vi "Func-Hex array string to bin file.vi"() -> ()   [LabVIEW 2015]
panel:
  out "array 2d":u8[][](array[numeric])=[[27, 0, 0, 0, 0, 0, 0, 0, 0, 0, 1, 56, 33, 80, 255, 239], [240, 93, 1, 0, 0, 0, 6, 1, 1, 165, 16, 0, 0, 2, 2, 2], [4, 4, 4, 4, 4, 4, 4, 0, 33, 191, 136, 2, 32, 32, 160, 132], [0, 6, 46, 47, 7, 211, 145, 27, 40, 68, 0, 10, 15, 0, 15, 108], [204, 91, 248, 23, 35, 154, 71, 0, 48, 24, 22, 108, 3, 96, 145, 2], [14, 120, 86, 16, 234, 42, 0, 31, 65, 0, 0, 0, 205, 124, 10, 137], [6, 8, 8, 3, 245, 0, 0, 39, 15, 128, 0, 128, 0, 0, 0, 0], [0, 255, 100, 100, 24, 1, 137, 6, 8, 8, 3, 245, 0, 0, 39, 15], [128, 0, 128, 0, 0, 0, 0, 0, 255, 100, 100, 24, 2, 137, 6, 8], [8, 3, 245, 0, 0, 39, 15, 128, 0, 128, 0, 0, 0, 0, 0, 255], [100, 100, 24, 3, 137, 6, 8, 8, 3, 245, 0, 0, 39, 15, 128, 0], [128, 0, 0, 0, 0, 0, 255, 100, 100, 24, 4, 137, 6, 8, 8, 3], [245, 0, 0, 39, 15, 128, 0, 128, 0, 0, 0, 0, 0, 255, 100, 100], [24, 5, 137, 6, 8, 8, 3, 245, 0, 0, 39, 15, 128, 0, 128, 0], [0, 0, 0, 0, 255, 100, 100, 24, 6, 137, 6, 8, 8, 3, 245, 0], [0, 39, 15, 128, 0, 128, 0, 0, 0, 0, 0, 255, 100, 100, 24, 7], [137, 6, 8, 8, 3, 245, 0, 0, 39, 15, 128, 0, 128, 0, 0, 0], [0, 0, 255, 100, 100, 24, 8, 137, 6, 8, 8, 3, 245, 0, 0, 39], [15, 128, 0, 128, 0, 0, 0, 0, 0, 255, 100, 100, 24, 9, 137, 6], [8, 8, 3, 245, 0, 0, 39, 15, 128, 0, 128, 0, 0, 0, 0, 0], [255, 100, 100, 24, 10, 137, 6, 8, 8, 3, 245, 0, 0, 39, 15, 128], [0, 128, 0, 0, 0, 0, 0, 255, 100, 100, 24, 11, 137, 6, 8, 8], [3, 245, 0, 0, 39, 15, 128, 0, 128, 0, 0, 0, 0, 0, 255, 100], [100, 24, 12, 137, 6, 8, 8, 3, 245, 0, 0, 39, 15, 128, 0, 128], [0, 0, 0, 0, 0, 255, 100, 100, 24, 13, 137, 6, 8, 8, 3, 245], [0, 0, 39, 15, 128, 0, 128, 0, 0, 0, 0, 0, 255, 100, 100, 24], [14, 137, 6, 8, 8, 3, 245, 0, 0, 39, 15, 128, 0, 128, 0, 0], [0, 0, 0, 255, 100, 100, 24, 15, 137, 6, 8, 8, 3, 245, 0, 0], [39, 15, 128, 0, 128, 0, 0, 0, 0, 0, 255, 100, 100, 24, 16, 137], [6, 8, 8, 3, 245, 0, 0, 39, 15, 128, 0, 128, 0, 0, 0, 0], [0, 255, 100, 100, 24, 17, 137, 6, 8, 8, 3, 245, 0, 0, 39, 15], [128, 0, 128, 0, 0, 0, 0, 0, 255, 100, 100, 24, 18, 128, 0, 0]] format="%02x"
  in  "Hex array string":string="1B\t00\t00\t00\t00\t00\t00\t00\t00\t00\t01\t38\t21\t50\tFF\tEF\nF0\t5D\t01\t00\t00\t00\t06\t01\t01\tA5\t10\t00\t00\t02\t02\t02\n04\t04\t04\t04\t04\t04\t04\t00\t21\tBF\t88\t02\t20\t20\tA0\t84\n00\t06\t2E\t2F\t07\tD3\t91\t1B\t28\t44\t00\t0A\t0F\t00\t0F\t6C\nCC\t5B\tF8\t17\t23\t9A\t47\t00\t30\t18\t16\t6C\t03\t60\t91\t02\n0E\t78\t56\t10\tEA\t2A\t00\t1F\t41\t00\t00\t00\tCD\t7C\t0A\t89\n06\t08\t08\t03\tF5\t00\t00\t27\t0F\t80\t00\t80\t00\t00\t00\t00\n00\tFF\t64\t64\t18\t01\t89\t06\t08\t08\t03\tF5\t00\t00\t27\t0F\n80\t00\t80\t00\t00\t00\t00\t00\tFF\t64\t64\t18\t02\t89\t06\t08\n08\t03\tF5\t00\t00\t27\t0F\t80\t00\t80\t00\t00\t00\t00\t00\tFF\n64\t64\t18\t03\t89\t06\t08\t08\t03\tF5\t00\t00\t27\t0F\t80\t00\n80\t00\t00\t00\t00\t00\tFF\t64\t64\t18\t04\t89\t06\t08\t08\t03\nF5\t00\t00\t27\t0F\t80\t00\t80\t00\t00\t00\t00\t00\tFF\t64\t64\n18\t05\t89\t06\t08\t08\t03\tF5\t00\t00\t27\t0F\t80\t00\t80\t00\n00\t00\t00\t00\tFF\t64\t64\t18\t06\t89\t06\t08\t08\t03\tF5\t00\n00\t27\t0F\t80\t00\t80\t00\t00\t00\t00\t00\tFF\t64\t64\t18\t07\n89\t06\t08\t08\t03\tF5\t00\t00\t27\t0F\t80\t00\t80\t00\t00\t00\n00\t00\tFF\t64\t64\t18\t08\t89\t06\t08\t08\t03\tF5\t00\t00\t27\n0F\t80\t00\t80\t00\t00\t00\t00\t00\tFF\t64\t64\t18\t09\t89\t06\n08\t08\t03\tF5\t00\t00\t27\t0F\t80\t00\t80\t00\t00\t00\t00\t00\nFF\t64\t64\t18\t0A\t89\t06\t08\t08\t03\tF5\t00\t00\t27\t0F\t80\n00\t80\t00\t00\t00\t00\t00\tFF\t64\t64\t18\t0B\t89\t06\t08\t08\n03\tF5\t00\t00\t27\t0F\t80\t00\t80\t00\t00\t00\t00\t00\tFF\t64\n64\t18\t0C\t89\t06\t08\t08\t03\tF5\t00\t00\t27\t0F\t80\t00\t80\n00\t00\t00\t00\t00\tFF\t64\t64\t18\t0D\t89\t06\t08\t08\t03\tF5\n00\t00\t27\t0F\t80\t00\t80\t00\t00\t00\t00\t00\tFF\t64\t64\t18\n0E\t89\t06\t08\t08\t03\tF5\t00\t00\t27\t0F\t80\t00\t80\t00\t00\n00\t00\t00\tFF\t64\t64\t18\t0F\t89\t06\t08\t08\t03\tF5\t00\t00\n27\t0F\t80\t00\t80\t00\t00\t00\t00\t00\tFF\t64\t64\t18\t10\t89\n06\t08\t08\t03\tF5\t00\t00\t27\t0F\t80\t00\t80\t00\t00\t00\t00\n00\tFF\t64\t64\t18\t11\t89\t06\t08\t08\t03\tF5\t00\t00\t27\t0F\n80\t00\t80\t00\t00\t00\t00\t00\tFF\t64\t64\t18\t12\t80\t00\t00"
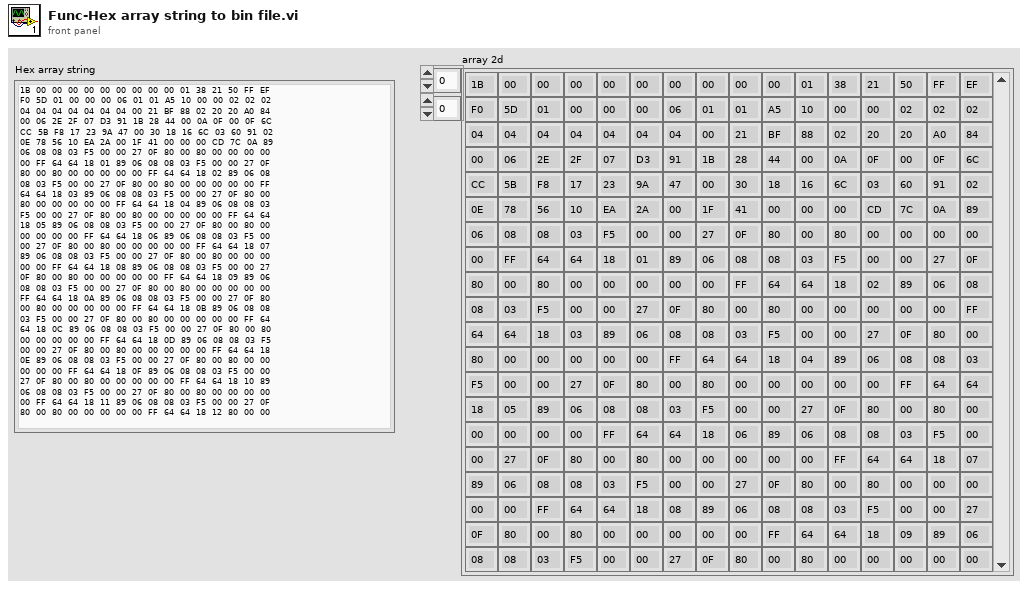
[diagram p1: front panel]
types:
  T1 = enum16{"open", "replace", "create", "open or create", "replace or create", "replace or create with confirmation"}
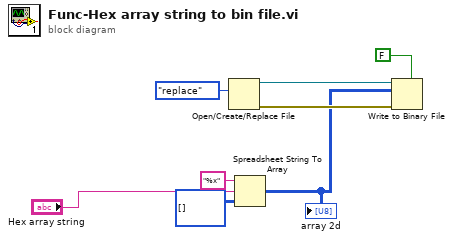
[diagram p0: block diagram]
diagram:
  n1 = Open/Create/Replace File(operation (0:open)=T1."replace" ("동작(0:open)")) -> (refnum out=w7:refnum<file>, error out=w6:errorcluster)  [unwired: 5 in, 1 out]
  n2 = Spreadsheet String To Array(format string="%x" ("포맷 문자열"), spreadsheet string="Hex array string", array type (2D Dbl)=u8[][] [] ("배열 타입(2D Dbl)")) -> (array=w2:u8[][])  [unwired: 1 in]
  "array 2d" <- w2
  n3 = Write to Binary File(file (use dialog)=w7, data=w2, error in=w6, 5:FALSE ("배열 또는 문자열 크기를 앞에 추가? (참)")) -> ()  [unwired: 2 in, 3 out]
